vi "race.vi"() -> ()   [LabVIEW 2019]
panel:
  in  "Numeric 3":dbl
  out "Numeric 2":dbl
  in  "Numeric":dbl
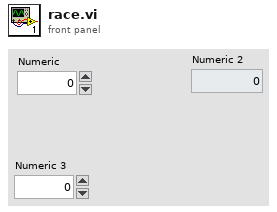
[diagram p1: front panel]
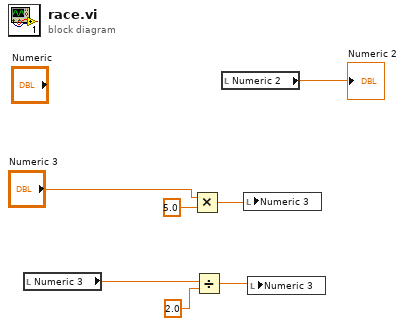
[diagram p0: block diagram]
diagram:
  n1 = local read "Numeric 3"() -> (w3:dbl)
  n2 = Multiply(x="Numeric 3", y=5.0) -> (x*y=w4:dbl)
  n3 = Divide(x=w3, y=2.0) -> (x/y=w1:dbl)
  n4 = local read "Numeric 2"() -> (→"Numeric 2":dbl)
  n5 = local write "Numeric 3"(w4) -> ()
  n6 = local write "Numeric 3"(w1) -> ()
